vi "solar_qtimer Destroy.vi"(8 "error in (no error)":errorcluster) -> (0 "error out":errorcluster)   [LabVIEW 2018]
doc: "[DEPRECIATED] This destroys all registered QTimers."
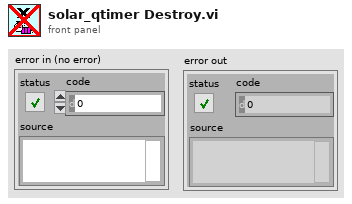
[diagram p1: front panel]
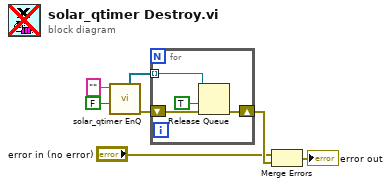
[diagram p0: block diagram]
diagram:
  n1 = call "solar_qtimer EnQ.vi"("Create if not found? (F)"=FALSE, "QTimer Name"="") -> ("error out"=w7:errorcluster, "All QTimers"=w3:refnum<queue>[])  [unwired: 7 in, 1 out]
  n2 = for {
    tunnel: w3 -> [w9] mode=indexing
    shift-right: [w10] -> w6
    shift-left: w7 -> [w11]
    n3 = Release Queue(queue=w9, force destroy? (F)=TRUE, error in (no error)=w11) -> (error out=w10:errorcluster)  [unwired: 2 out]
  }
  n4 = Merge Errors("error in (no error)", w6) -> (→"error out":errorcluster)
